vi "circle-area-perimeter_2.vi"() -> ()   [LabVIEW 2025]
panel:
  in  "CL":bool
  in  "2":bool
  out "?":string
  in  "OK":bool
  in  "1 .":bool
  in  "0":bool
  in  "9":bool
  in  "8":bool
  in  "7":bool
  in  "6":bool
  in  "5":bool
  in  "4":bool
  in  "3":bool
  in  "1":bool
  in  "stop":bool
  out "Area":dbl
  out "Perimeter":dbl
  # "Enter Radius"
  # "1"
  # "2"
  # "3"
  # "4"
  # "5"
  # "6"
  # "7"
  # "8"
  # "9"
  # "."
  # "0"
  # "CL"
  # "OK"
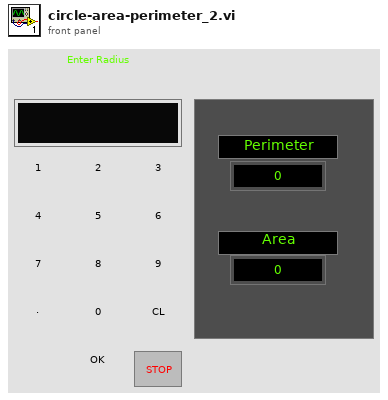
[diagram p1: front panel]
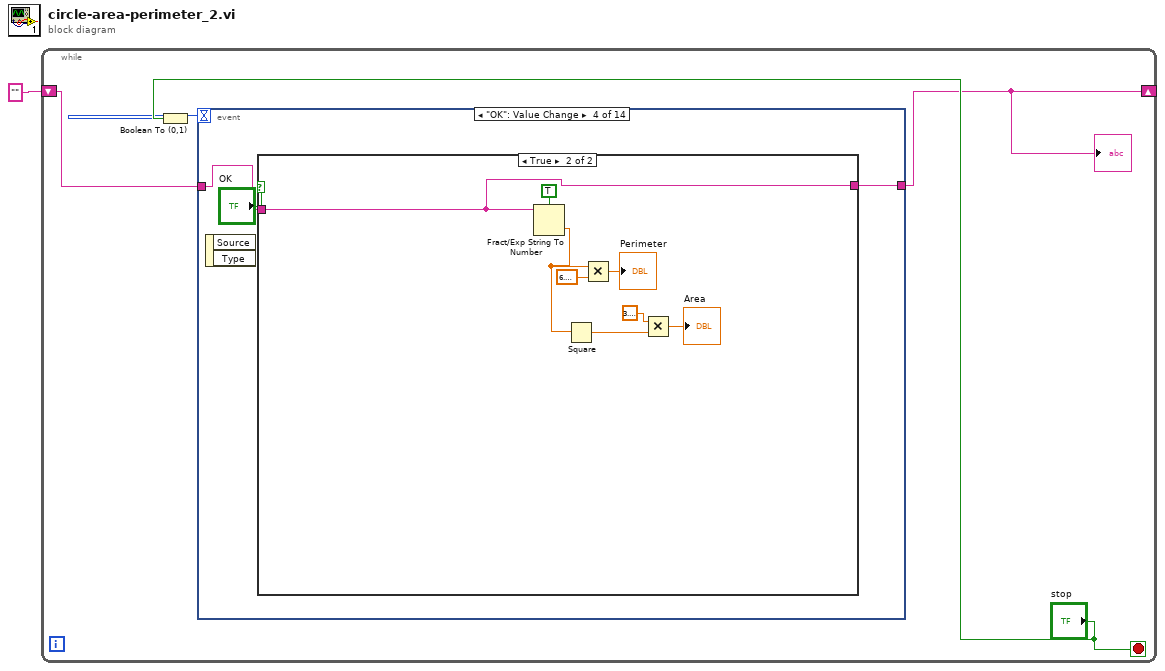
[diagram p0: block diagram]
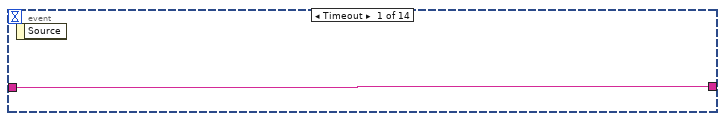
[diagram p2: hidden frame]
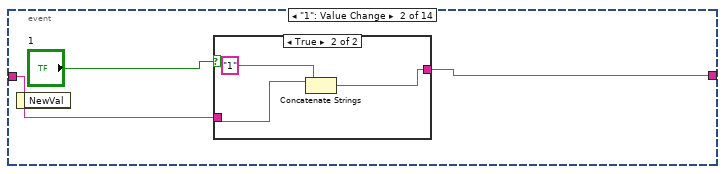
[diagram p3: hidden frame]
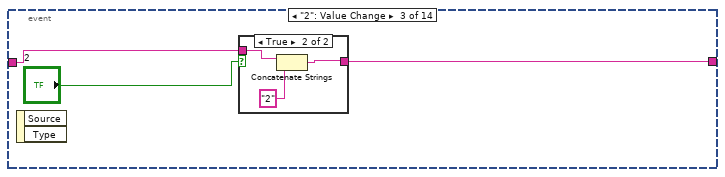
[diagram p5: hidden frame]
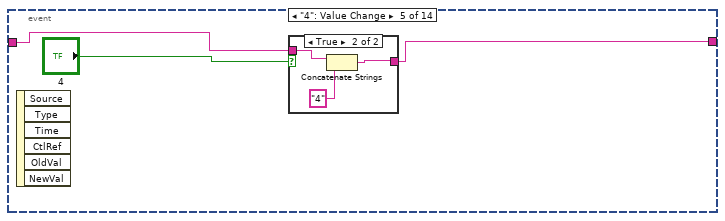
[diagram p8: hidden frame]
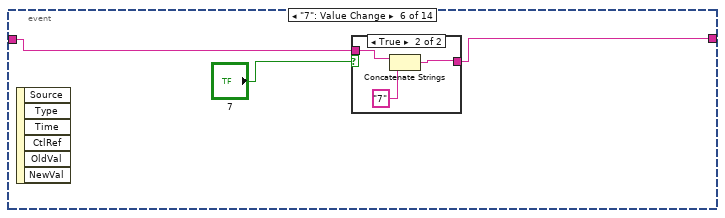
[diagram p10: hidden frame]
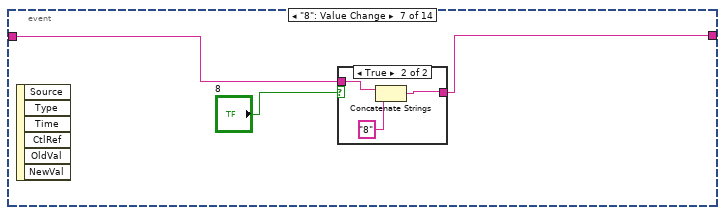
[diagram p12: hidden frame]
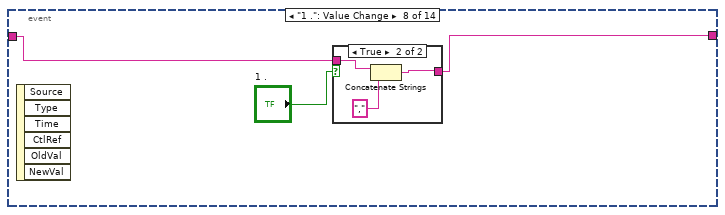
[diagram p14: hidden frame]
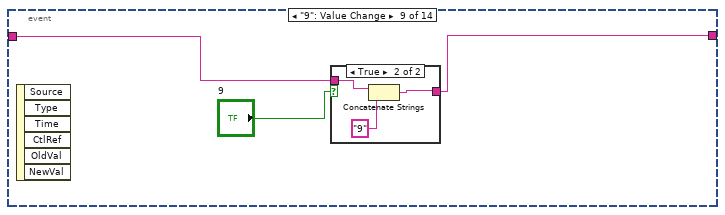
[diagram p16: hidden frame]
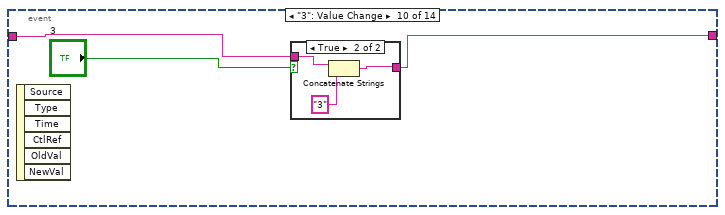
[diagram p18: hidden frame]
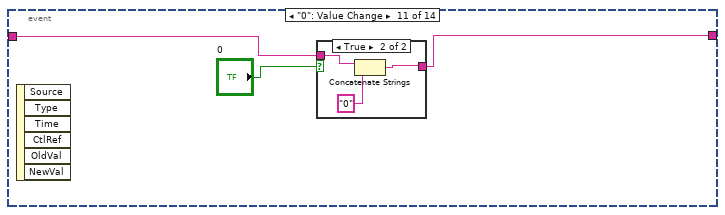
[diagram p20: hidden frame]
diagram:
  n1 = while {
    shift-right: [w2] -> _
    shift-left: "" -> [w5]
    stop <- "stop" stop-if-true
    n2 = Boolean To (0,1)(Boolean="stop") -> (0, 1=w3:i16)
    n3 = event shown="[3] \"OK\": Value Change" {
      selector: _ -> [_ _ _ _ _ _ _ _ _ _ _ _ _ _]
      dyn-events: _ -> [_ _ _ _ _ _ _ _ _ _ _ _ _ _]
      timeout: w3 -> [_ _ _ _ _ _ _ _ _ _ _ _ _ _]
      tunnel: [w6 w7 w14 w21 w33 w40 w47 w54 w61 w68 w75 w82 w89 w96] -> w2
      tunnel: w5 -> [w6 w8 w15 w22 w34 w41 w48 w55 w62 w69 w76 w83 w90 w97]
      event Timeout {
        n4 = event-data() -> ()  [unwired: 1 in, 1 out]
      }
      event "1": Value Change {
        n5 = event-data() -> ()  [unwired: 1 in, 1 out]
        n6 = case shown="True" "1" {
          tunnel: w8 -> [w10 w13]
          tunnel: [w10 w12] -> w7
          frame False {
          }
          frame True {
            n7 = Concatenate Strings(w13, "1") -> (w12:string)
          }
        }
      }
      event "2": Value Change {
        n8 = event-data() -> ()  [unwired: 1 in, 2 out]
        n9 = case shown="True" "2" {
          tunnel: [w17 w20] -> w14
          tunnel: w15 -> [w17 w18]
          frame False {
          }
          frame True {
            n10 = Concatenate Strings(w18, "2") -> (w20:string)
          }
        }
      }
      event "OK": Value Change {
        n11 = event-data() -> ()  [unwired: 1 in, 2 out]
        n12 = case shown="True" "OK" {
          tunnel: w22 -> [w24 w25]
          tunnel: [w24 w25] -> w21
          frame False {
          }
          frame True {
            n13 = Fract/Exp String To Number(use system decimal point (T)=TRUE, string=w25) -> (number=w26:dbl)  [unwired: 2 in, 1 out]
            n14 = Square(x=w26) -> (x^2=w29:dbl)
            n15 = Multiply(x=w26, y=6.283185307179586) -> (x*y=→"Perimeter":dbl)
            n16 = Multiply(x=3.141592653589793, y=w29) -> (x*y=→"Area":dbl)
          }
        }
      }
      event "4": Value Change {
        n17 = event-data() -> ()  [unwired: 1 in, 6 out]
        n18 = case shown="True" "4" {
          tunnel: [w36 w39] -> w33
          tunnel: w34 -> [w36 w37]
          frame False {
          }
          frame True {
            n19 = Concatenate Strings(w37, "4") -> (w39:string)
          }
        }
      }
      event "7": Value Change {
        n20 = event-data() -> ()  [unwired: 1 in, 6 out]
        n21 = case shown="True" "7" {
          tunnel: [w43 w46] -> w40
          tunnel: w41 -> [w43 w44]
          frame False {
          }
          frame True {
            n22 = Concatenate Strings(w44, "7") -> (w46:string)
          }
        }
      }
      event "8": Value Change {
        n23 = event-data() -> ()  [unwired: 1 in, 6 out]
        n24 = case shown="True" "8" {
          tunnel: [w50 w53] -> w47
          tunnel: w48 -> [w50 w51]
          frame False {
          }
          frame True {
            n25 = Concatenate Strings(w51, "8") -> (w53:string)
          }
        }
      }
      event "1 .": Value Change {
        n26 = event-data() -> ()  [unwired: 1 in, 6 out]
        n27 = case shown="True" "1 ." {
          tunnel: [w57 w60] -> w54
          tunnel: w55 -> [w57 w58]
          frame False {
          }
          frame True {
            n28 = Concatenate Strings(w58, ",") -> (w60:string)
          }
        }
      }
      event "9": Value Change {
        n29 = event-data() -> ()  [unwired: 1 in, 6 out]
        n30 = case shown="True" "9" {
          tunnel: [w64 w67] -> w61
          tunnel: w62 -> [w64 w65]
          frame False {
          }
          frame True {
            n31 = Concatenate Strings(w65, "9") -> (w67:string)
          }
        }
      }
      event "3": Value Change {
        n32 = event-data() -> ()  [unwired: 1 in, 6 out]
        n33 = case shown="True" "3" {
          tunnel: [w71 w74] -> w68
          tunnel: w69 -> [w71 w72]
          frame False {
          }
          frame True {
            n34 = Concatenate Strings(w72, "3") -> (w74:string)
          }
        }
      }
      event "0": Value Change {
        n35 = event-data() -> ()  [unwired: 1 in, 6 out]
        n36 = case shown="True" "0" {
          tunnel: [w78 w81] -> w75
          tunnel: w76 -> [w78 w79]
          frame False {
          }
          frame True {
            n37 = Concatenate Strings(w79, "0") -> (w81:string)
          }
        }
      }
      event "5": Value Change {
        n38 = event-data() -> ()  [unwired: 1 in, 6 out]
        n39 = case shown="True" "5" {
          tunnel: [w85 w88] -> w82
          tunnel: w83 -> [w85 w86]
          frame False {
          }
          frame True {
            n40 = Concatenate Strings(w86, "5") -> (w88:string)
          }
        }
      }
      event "6": Value Change {
        n41 = event-data() -> ()  [unwired: 1 in, 6 out]
        n42 = case shown="True" "6" {
          tunnel: [w92 w95] -> w89
          tunnel: w90 -> [w92 w93]
          frame False {
          }
          frame True {
            n43 = Concatenate Strings(w93, "6") -> (w95:string)
          }
        }
      }
      event "CL": Value Change {
        n44 = event-data() -> ()  [unwired: 1 in, 6 out]
        n45 = case shown="True" "CL" {
          tunnel: [w99 ""] -> w96
          tunnel: w97 -> [w99 _]
          frame False {
          }
          frame True {
          }
        }
      }
    }
    "?" <- w2
  }
